vi "Boiler.vi"() -> ()   [LabVIEW 2023]
uses:
  Controls/Boiler Controls.ctl
  Controls/Boiler Simulation Controls.ctl
  Controls/Boiler Status Indicators.ctl
  Controls/State.ctl
  Controls/DataCluster.ctl
panel:
  out "error out":errorcluster
  in  "error in (no error)":errorcluster
  in  "stop":bool
  out "Boiler Status Indicators":T1={"Status"="Lockout", "Primary Fan"=FALSE, "Natural Gas Valve"=FALSE, "Pilot"=FALSE, "Fuel Valve"=FALSE, "Forced Draft Fan"=FALSE, "Time Count"=0.0} {"Time Count" format="%.2g"}
  in  "Boiler Simulation Controls":T2 {"Flame Sensor Value (%)" min=0.0 max=100.0 scale=0.0..100.0}
  in  "Boiler Controls":T3 {"Fuel Valve Position" min=0.0 max=100.0 scale=0.0..100.0 scale format="%.2f"}
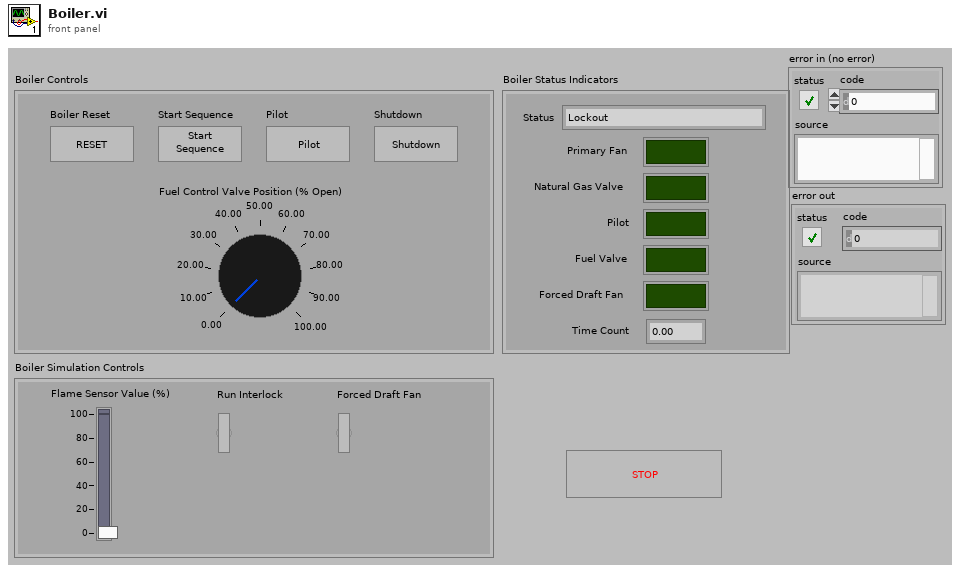
[diagram p1: front panel]
types:
  T1 = typedef "Boiler Status Indicators.ctl" = cluster{"Status":string, "Primary Fan":bool, "Natural Gas Valve":bool, "Pilot":bool, "Fuel Valve":bool, "Forced Draft Fan":bool, "Time Count":dbl}
  T2 = typedef "Boiler Simulation Controls.ctl" = cluster{"Flame Sensor Value (%)":dbl, "Run Interlock":bool, "Forced Draft Fan":bool}
  T3 = typedef "Boiler Controls.ctl" = cluster{"Boiler Reset":bool, "Start Sequence":bool, "Pilot":bool, "Shutdown":bool, "Fuel Valve Position":dbl}
  T4 = typedef "DataCluster.ctl" = cluster{"Boiler Log Path":path, "Last State":T5, "Time out":i32, "Ini Values":cluster{"Timer Count":dbl, "Flame Range Value":dbl}, "Flame Sensor Val":dbl}
  T5 = typedef "State.ctl" = enum16{"Boiler Initialized", "Boiler Ready", "Start Pre-Purge", "Pre-Purge Complete", "Pilot On", "Pilot Proved", "Force Draft Fan ON", "Shutdown and Purge", "Wait for Something"}
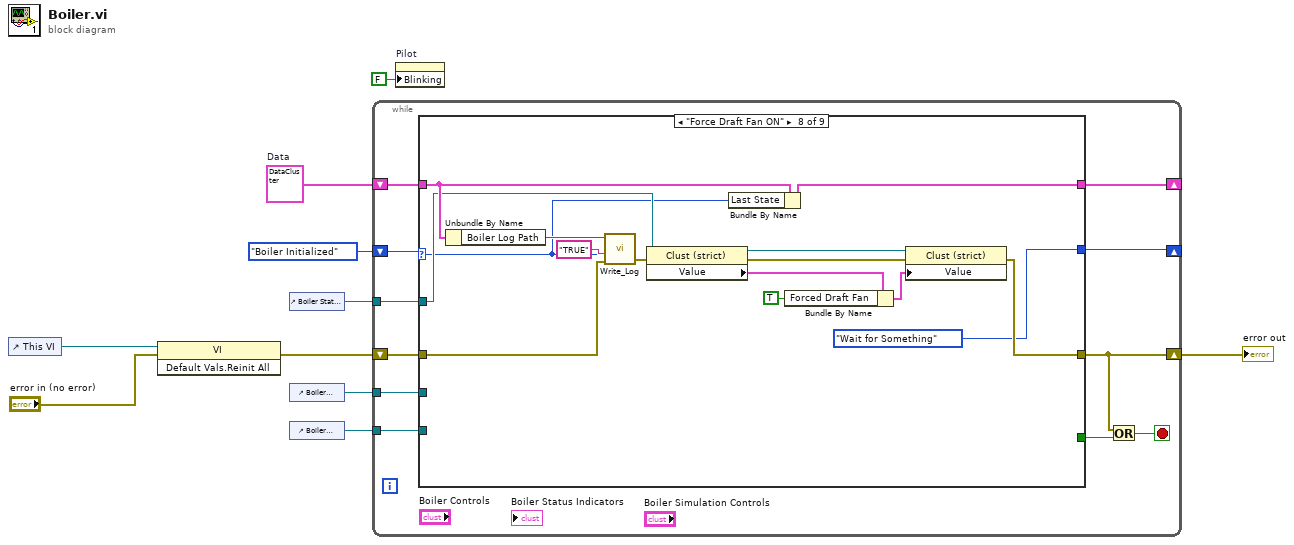
[diagram p0: block diagram]
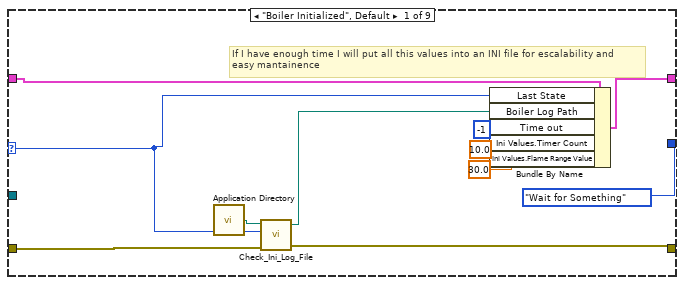
[diagram p2: hidden frame]
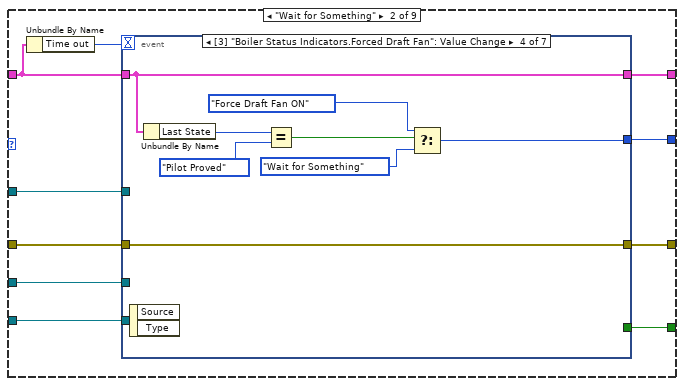
[diagram p3: hidden frame]
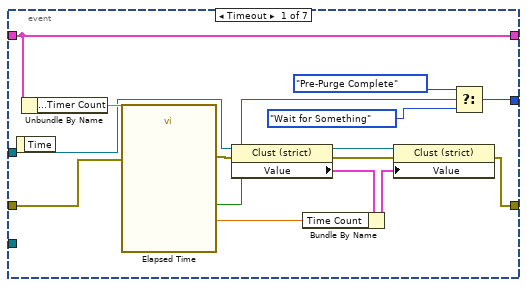
[diagram p4: hidden frame]
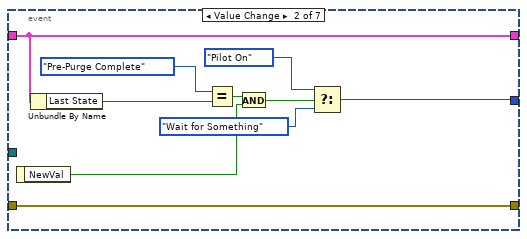
[diagram p5: hidden frame]
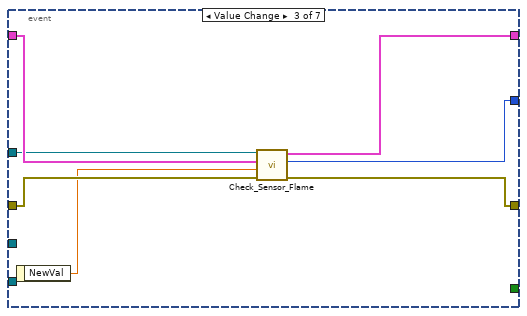
[diagram p6: hidden frame]
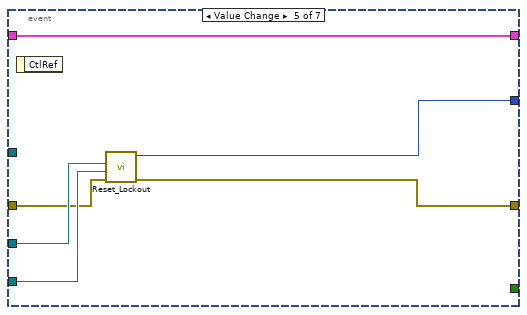
[diagram p7: hidden frame]
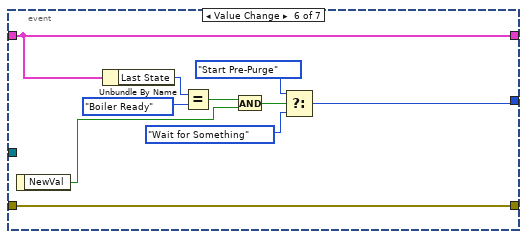
[diagram p8: hidden frame]
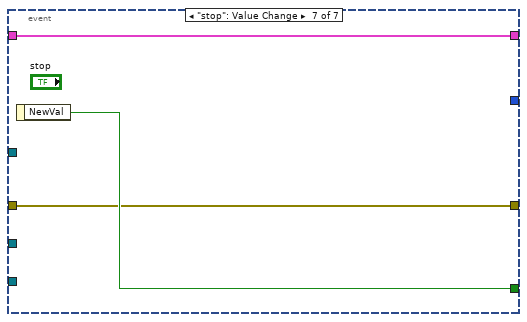
[diagram p9: hidden frame]
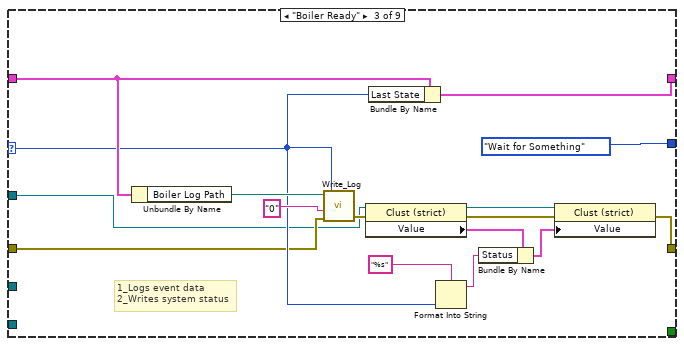
[diagram p10: hidden frame]
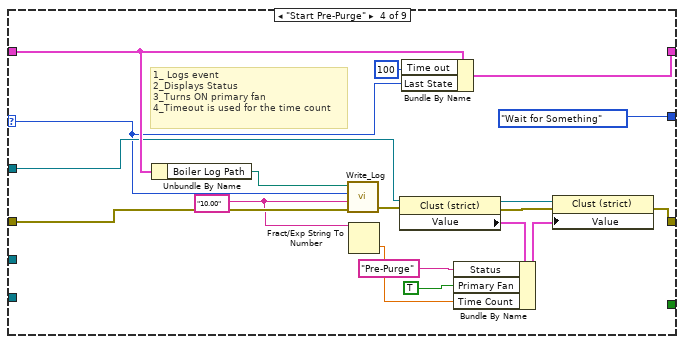
[diagram p11: hidden frame]
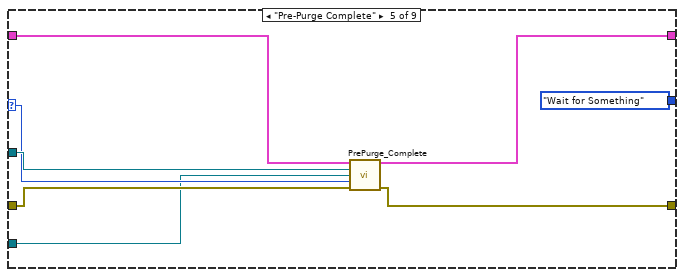
[diagram p12: hidden frame]
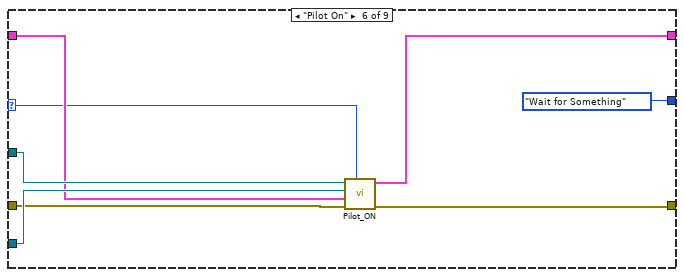
[diagram p13: hidden frame]
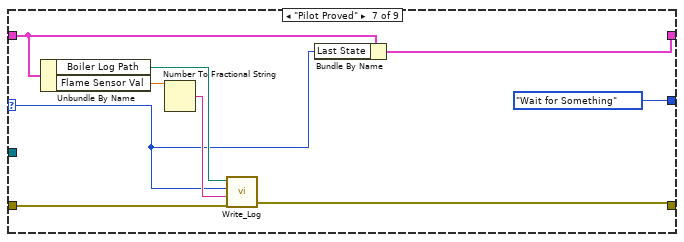
[diagram p14: hidden frame]
diagram:
  w5 = T4 {"Boiler Log Path"=path "", "Last State"=enum."Boiler Initialized", "Time out"=0, "Ini Values"={"Timer Count"=0.0, "Flame Range Value"=0.0}, "Flame Sensor Val"=0.0}  # Data
  n1 = control-ref of="This VI"() -> (w10:refnum<vi>)
  n2 = invoke class="VI" method="Default Vals.Reinit All"(reference=w10, error in="error in (no error)") -> (error out=w9:errorcluster)  [unwired: 1 in, 2 out]
  n3 = control-ref of="Boiler Status Indicators"() -> (w2:refnum<vi>)
  n4 = control-ref of="Boiler Controls"() -> (w4:refnum<vi>)
  n5 = control-ref of="Boiler Simulation Controls"() -> (w3:refnum<vi>)
  n6 = while {
    shift-right: [w20] -> w7
    shift-left: w9 -> [w21]
    shift-right: [w15] -> _
    shift-left: w5 -> [w16]
    shift-right: [w14] -> _
    shift-left: State."Boiler Initialized" -> [w17]
    tunnel: w4 -> [w13]
    tunnel: w3 -> [w12]
    tunnel: w2 -> [w11]
    stop <- w19 stop-if-true
    n7 = case shown="\"Force Draft Fan ON\"" w17 {
      selector: w17 -> [w26 _ w107 w118 w138 w144 w152 w162 _]
      tunnel: w21 -> [w31 w42 w106 w131 w142 w148 w160 w175 w177]
      tunnel: [w30 w41 w103 w122 w140 w146 w159 w168 w177] -> w20
      tunnel: [_ w40 _ _ _ _ _ _ _] -> w18
      tunnel: w16 -> [w32 w34 w114 w135 w143 w147 w158 w173 w176]
      tunnel: [w27 w35 w117 w120 w139 w145 w153 w163 w176] -> w15
      tunnel: [State."Wait for Something" w36 State."Wait for Something" ("State Out") State."Wait for Something" ("State Out") State."Wait for Something" ("State Out") State."Wait for Something" ("State Out") State."Wait for Something" ("State Out") State."Wait for Something" ("State Out") _] -> w14
      tunnel: w13 -> [_ w39 _ _ w137 w150 _ _ _]
      tunnel: w12 -> [_ w38 _ _ _ _ _ _ _]
      tunnel: w11 -> [_ w37 w102 w133 w141 w149 _ w169 _]
      frame "Boiler Initialized", Default {
        # "If I have enough time I will put all this values into an INI file for escalability and\neasy mantainence"
        n8 = call <vilib>:"Application Directory.vi"() -> ("Application Directory"=w29:path)
        n9 = call "Check_Ini_Log_File.vi"("Application path"=w29, "State"=w26, "error in (no error)"=w31) -> ("Application path"=w25:path, "error out"=w30:errorcluster)  [unwired: 3 in]
        n10 = Bundle By Name(cluster=w32, "Last State"=w26, "Boiler Log Path"=w25, "Time out"=-1, "Ini Values.Timer Count"=10.0 ("Timer Count"), "Ini Values.Flame Range Value"=30.0 ("Ini Values.Flame Value")) -> (w27:T4)
      }
      frame "Wait for Something" {
        n11 = Unbundle By Name(w34) -> ("Time out"=w33:i32)
        n12 = event shown="[3] \"Boiler Status Indicators.Forced Draft Fan\": Value Change" {
          selector: _ -> [_ _ _ _ _ _ _]
          dyn-events: _ -> [_ _ _ _ _ _ _]
          timeout: w33 -> [_ _ _ _ _ _ _]
          tunnel: w42 -> [w57 w67 w74 w76 w86 w98 w100]
          tunnel: [w50 w67 w71 w76 w85 w98 w100] -> w41
          tunnel: [_ _ _ _ _ _ w101] -> w40
          tunnel: w39 -> [_ _ _ _ w88 _ _]
          tunnel: w38 -> [_ _ _ _ w87 _ _]
          tunnel: w37 -> [w53 _ w72 _ _ _ _]
          tunnel: [w44 w60 w70 w78 w84 w91 _] -> w36
          tunnel: w34 -> [w55 w66 w73 w82 w83 w96 w99]
          tunnel: [w55 w66 w69 w82 w83 w96 w99] -> w35
          event Timeout {
            n13 = event-data() -> ()  [unwired: 1 in, 1 out]
            n14 = Unbundle By Name(w55) -> ("Ini Values.Timer Count"=w54:dbl)
            n15 = call "Elapsed Time"("Time Target (s)"=w54, "error in (no error)"=w57) -> ("Elapsed Time (s)"=w47:dbl, "Time has Elapsed"=w46:bool, "error out"=w56:errorcluster)  [unwired: 10 in, 5 out]
            n16 = property class="Clust (strict)"(reference=w53, error in=w56) -> (reference out=w52:refnum<vi>, error out=w51:errorcluster, "Value"=w49:T1)
            n17 = Bundle By Name(cluster=w49, "Time Count"=w47) -> (w48:T1)
            n18 = property class="Clust (strict)"(reference=w52, error in=w51, "Value"=w48) -> (error out=w50:errorcluster)  [unwired: 1 out]
            n19 = Select(t=State."Pre-Purge Complete", s=w46, f=State."Wait for Something") -> (s? t:f=w44:T5)
          }
          event Value Change {
            n20 = event-data() -> ("NewVal"=w62:bool)  [unwired: 1 in]
            n21 = Unbundle By Name(w66) -> ("Last State"=w65:T5)
            n22 = Equal?(x=State."Pre-Purge Complete", y=w65) -> (x = y?=w63:bool)
            n23 = And(x=w63, y=w62) -> (x .and. y?=w61:bool)
            n24 = Select(t=State."Pilot On" ("x"), s=w61, f=State."Wait for Something" ("x")) -> (s? t:f=w60:T5)
          }
          event Value Change {
            n25 = event-data() -> ("NewVal"=w68:dbl)  [unwired: 1 in]
            n26 = call "Check_Sensor_Flame.vi"("error in (no error)"=w74, "NewVal"=w68, "Data in"=w73, "Cluster in"=w72) -> ("error out"=w71:errorcluster, "State"=w70:T5, "Data out"=w69:T4)  [unwired: 5 in]
          }
          event Value Change {
            n27 = event-data() -> ()  [unwired: 1 in, 2 out]
            n28 = Unbundle By Name(w82) -> ("Last State"=w81:T5)
            n29 = Equal?(x=w81, y=State."Pilot Proved") -> (x = y?=w79:bool)
            n30 = Select(t=State."Force Draft Fan ON" ("y"), s=w79, f=State."Wait for Something" ("y")) -> (s? t:f=w78:T5)
          }
          event Value Change {
            n31 = event-data() -> ()  [unwired: 1 in, 1 out]
            n32 = call "Reset_Lockout.vi"("error in (no error)"=w86, "Boiler Simulation Controls"=w87, "Boiler Controls"=w88) -> ("error out"=w85:errorcluster, "State Out"=w84:T5)  [unwired: 3 in]
          }
          event Value Change {
            n33 = event-data() -> ("NewVal"=w97:bool)  [unwired: 1 in]
            n34 = Unbundle By Name(w96) -> ("Last State"=w95:T5)
            n35 = Equal?(x=w95, y=State."Boiler Ready") -> (x = y?=w93:bool)
            n36 = And(x=w93, y=w97) -> (x .and. y?=w92:bool)
            n37 = Select(t=State."Start Pre-Purge", s=w92, f=State."Wait for Something") -> (s? t:f=w91:T5)
          }
          event "stop": Value Change {
            n38 = event-data() -> ("NewVal"=w101:bool)  [unwired: 1 in]
          }
        }
      }
      frame "Boiler Ready" {
        # "1_Logs event data\n2_Writes system status"
        n39 = Unbundle By Name(w114) -> ("Boiler Log Path"=w113:path)
        n40 = call "Write_Log.vi"("error in (no error)"=w106, "Event data string"="0", "State"=w107, "dup path"=w113) -> ("error out"=w105:errorcluster)  [unwired: 2 in]
        n41 = property class="Clust (strict)"(reference=w102, error in=w105) -> (reference out=w110:refnum<vi>, error out=w104:errorcluster, "Value"=w109:T1)
        n42 = Bundle By Name(cluster=w114, "Last State"=w107) -> (w117:T4)
        n43 = Format Into String(format string="%s", w107) -> (resulting string=w112:string)  [unwired: 2 in, 1 out]
        n44 = Bundle By Name(cluster=w109, "Status"=w112) -> (w108:T1)
        n45 = property class="Clust (strict)"(reference=w110, error in=w104, "Value"=w108) -> (error out=w103:errorcluster)  [unwired: 1 out]
      }
      frame "Start Pre-Purge" {
        w125 = "10.00"
        # "1_ Logs event\n2_Displays Status\n3_Turns ON primary fan\n4_Timeout is used for the time count"
        n46 = Unbundle By Name(w135) -> ("Boiler Log Path"=w134:path)
        n47 = call "Write_Log.vi"("error in (no error)"=w131, "Event data string"=w125, "State"=w118, "dup path"=w134) -> ("error out"=w123:errorcluster)  [unwired: 2 in]
        n48 = Fract/Exp String To Number(string=w125) -> (number=w124:dbl)  [unwired: 3 in, 1 out]
        n49 = property class="Clust (strict)"(reference=w133, error in=w123) -> (reference out=w132:refnum<vi>, error out=w130:errorcluster, "Value"=w129:T1)
        n50 = Bundle By Name(cluster=w135, "Time out"=100, "Last State"=w118) -> (w120:T4)
        n51 = Bundle By Name(cluster=w129, "Status"="Pre-Purge", "Primary Fan"=TRUE, "Time Count"=w124) -> (w128:T1)
        n52 = property class="Clust (strict)"(reference=w132, error in=w130, "Value"=w128) -> (error out=w122:errorcluster)  [unwired: 1 out]
      }
      frame "Pre-Purge Complete" {
        n53 = call "PrePurge_Complete.vi"("Data in"=w143, "Boiler Status Indicators"=w141, "Boiler Controls"=w137, "State"=w138, "error in (no error)"=w142) -> ("Data out"=w139:T4, "error out"=w140:errorcluster)  [unwired: 9 in]
      }
      frame "Pilot On" {
        n54 = call "Pilot_ON.vi"("State"=w144, "error in (no error)"=w148, "Data in"=w147, 10:"Boiler Controls"=w150, 11:"Boiler Controls"=w149) -> ("error out"=w146:errorcluster, "Data out"=w145:T4)  [unwired: 5 in]
      }
      frame "Pilot Proved" {
        n55 = Unbundle By Name(w158) -> ("Boiler Log Path"=w157:path, "Flame Sensor Val"=w156:dbl)
        n56 = Number To Fractional String(number=w156) -> (F-format string=w155:string)  [unwired: 3 in]
        n57 = call "Write_Log.vi"("error in (no error)"=w160, "Event data string"=w155, "State"=w152, "dup path"=w157) -> ("error out"=w159:errorcluster)  [unwired: 2 in]
        n58 = Bundle By Name(cluster=w158, "Last State"=w152) -> (w153:T4)
      }
      frame "Force Draft Fan ON" {
        n59 = Unbundle By Name(w173) -> ("Boiler Log Path"=w172:path)
        n60 = call "Write_Log.vi"("error in (no error)"=w175, "Event data string"="TRUE", "State"=w162, "dup path"=w172) -> ("error out"=w174:errorcluster)  [unwired: 2 in]
        n61 = property class="Clust (strict)"(reference=w169, error in=w174) -> (reference out=w167:refnum<vi>, error out=w170:errorcluster, "Value"=w166:T1)
        n62 = Bundle By Name(cluster=w173, "Last State"=w162) -> (w163:T4)
        n63 = Bundle By Name(cluster=w166, "Forced Draft Fan"=TRUE) -> (w165:T1)
        n64 = property class="Clust (strict)"(reference=w167, error in=w170, "Value"=w165) -> (error out=w168:errorcluster)  [unwired: 1 out]
      }
      frame "Shutdown and Purge" {
      }
    }
    n65 = Or(x=w20, y=w18) -> (x .or. y?=w19:bool)
  }
  "error out" <- w7
  n66 = property on="Pilot" class="Bool (strict)"("Blinking"=FALSE) -> ()  [unwired: 2 in, 2 out]
